vi "ac2dc.vi"(2 "Pac":dbl format="%#_13g", 3 "eta [pu]":dbl format="%#_13g") -> (0 "Pdc":dbl format="%#_13g")   [LabVIEW 2021]
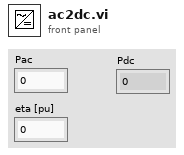
[diagram p1: front panel]
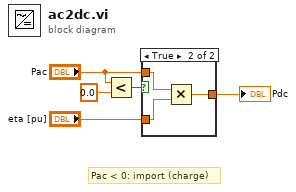
[diagram p0: block diagram]
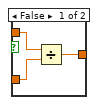
[diagram p2: hidden frame]
diagram:
  # "Pac < 0: import (charge)"
  n1 = Less?(x="Pac", y=0.0) -> (x < y?=w4:bool)
  n2 = case shown="True" w4 {
    tunnel: [w8 w9] -> w5
    tunnel: "Pac" -> [w7 w11]
    tunnel: "eta [pu]" -> [w6 w10]
    frame False {
      n3 = Divide(x=w7, y=w6) -> (x/y=w8:dbl)
    }
    frame True {
      n4 = Multiply(x=w11, y=w10) -> (x*y=w9:dbl)
    }
  }
  "Pdc" <- w5
